vi "Get Exported DTC Control.vi"(8 "error in (no error)":errorcluster, 11 "Section Ref in":T1 format="%.0x") -> (0 "error out":errorcluster, 2 "DTCControl":T2 {"Signals"."Byte Order" items=["Little Endian", "Big Endian"]; "Signals"."Data Type" items=["Signed", "Unsigned", "IEEE Float"]}, 3 "Section Ref out":T1 format="%.0x")   [LabVIEW 2015, in "Diagnostics Addon System Explorer.lvlib"]
uses:
  Diagnostics Addon System Explorer.lvlib
  Shared/Types/Exported DTC Control Cluster.ctl
  Shared/Types/Signal Parameters.ctl
  <vilib>/NI Veristand/Custom Device API/Custom Device Item Ref.ctl
  Types/FG Action.ctl
  Signal Parameters FG.vi
  <vilib>/NI Veristand/Custom Device API/NI VeriStand - Get Item Property.vi
  <vilib>/NI Veristand/Custom Device API/Get Item Property (U32).vi
  <vilib>/NI Veristand/Custom Device API/NI VeriStand - Set Item Property.vi
  <vilib>/NI Veristand/Custom Device API/Set Item Property (U32).vi
  Shared/SubVIs/GUID Lookup.vi
  <vilib>/NI Veristand/Custom Device API/NI VeriStand - Get Custom Device Channel Data.vi
  <vilib>/NI Veristand/Custom Device API/Get Item Property (String).vi
  <vilib>/NI Veristand/Custom Device API/Get Item Property (Double).vi
  <vilib>/NI Veristand/Custom Device API/Set Item Property (String).vi
  <vilib>/NI Veristand/Custom Device API/Set Item Property (Double).vi
  <vilib>/NI Veristand/Custom Device API/NI VeriStand - Get Item Children.vi
  <vilib>/NI Veristand/Custom Device Tools/Custom Device Utility Library/NI VeriStand - Search for Item by GUID.vi
  Shared/Diagnostics Addon Shared.lvlib
  <vilib>/NI Veristand/Custom Device Tools/Custom Device Utility Library/Custom Device Utility Library.lvlib
  <vilib>/NI Veristand/Custom Device API/Custom Device API.lvlib
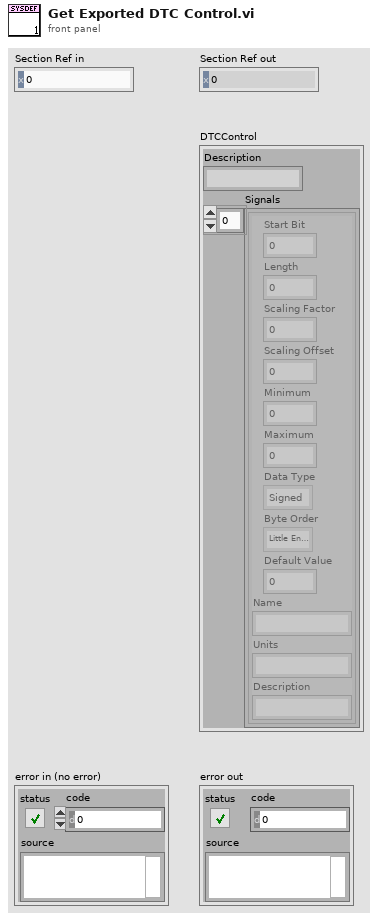
[diagram p1: front panel]
types:
  T1 = typedef "Custom Device API.lvlib/Custom Device Item Ref.ctl" = u64
  T2 = typedef "Diagnostics Addon Shared.lvlib/Exported DTC Control Cluster.ctl" = cluster{"Description":string, "Signals":T3[]}
  T3 = typedef "Diagnostics Addon Shared.lvlib/Signal Parameters.ctl" = cluster{"Start Bit":u8, "Length":u8, "Scaling Factor":dbl, "Scaling Offset":dbl, "Minimum":dbl, "Maximum":dbl, "Data Type":u32, "Byte Order":u32, "Default Value":dbl, "Name":string, "Units":string, "Description":string}
  T4 = typedef "Diagnostics Addon System Explorer.lvlib/FG Action.ctl" = enum16{"Get", "Set"}
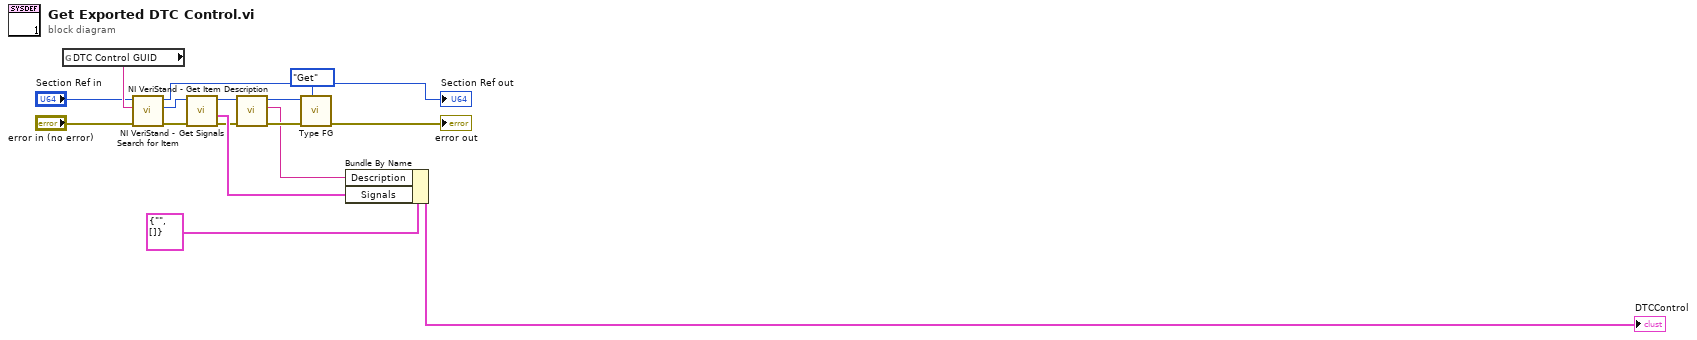
[diagram p0: block diagram]
diagram:
  n1 = global read "GUID Lookup.vi" "DTC Control GUID"() -> (w8:string)
  n2 = call-poly <vilib>:"NI VeriStand - Search for Item.vi"("error in"="error in (no error)", "Item GUID"=w8, "Section Ref in"="Section Ref in") -> ("error out"=w4:errorcluster, "Item Ref"=w3:T1, "Section Ref out"=→"Section Ref out":T1)  [unwired: 5 in, 1 out]
  n3 = call "Get Signals.vi"("error in (no error)"=w4, "Device Item Ref out"=w3) -> ("error out"=w5:errorcluster, "Parameters"=w11:T3[], "Item Ref out"=w6:T1)  [unwired: 6 in, 1 out]
  n4 = call <vilib>:"NI VeriStand - Get Item Description.vi"("error in (no error)"=w5, "Item Ref in"=w6) -> ("error out"=w14:errorcluster, "Description"=w10:string, "Item Ref out"=w16:T1)  [unwired: 7 out]
  n5 = call "Type FG.vi"("Action"=FG_Action."Get", "error in (no error)"=w14, "Device Item Ref in"=w16) -> ("error out"=→"error out":errorcluster)  [unwired: 6 in, 2 out]
  n6 = Bundle By Name(cluster=T2 {"Description"="", "Signals"=[]} ("DTCControl"), "Description"=w10, "Signals"=w11) -> (→"DTCControl":T2)
